vi "Get Column Object.vi"(8 "error in (no error)":errorcluster, 10 "Column Name":string, 11 "Table in":refnum<class "Table.lvclass">) -> (0 "error out":errorcluster, 2 "Column Object":refnum<class "Column Interface.lvclass">, 3 "Table out":refnum<class "Table.lvclass">)   [LabVIEW 2020, in "Table.lvlib" / "Table.lvclass"]
uses:
  Table.lvclass
  Column Interface/Column Interface Class/Column Interface.lvclass
  Table.lvclass/Table.ctl
  Table Configuration Interface/Table Configuration Interface.lvclass
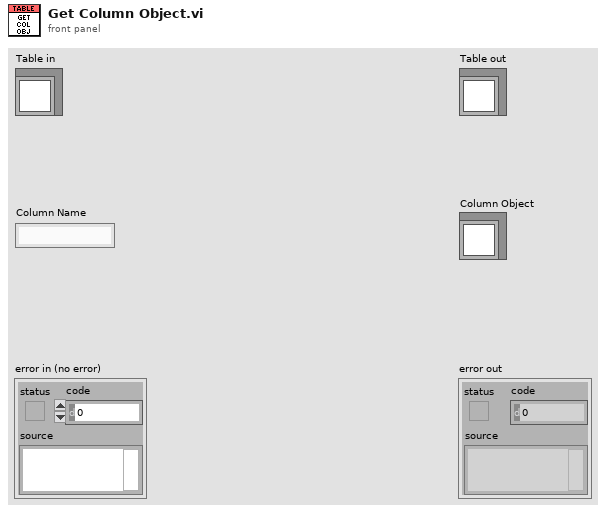
[diagram p1: front panel]
types:
  T1 = map{string, refnum<class "Column Interface.lvclass">}
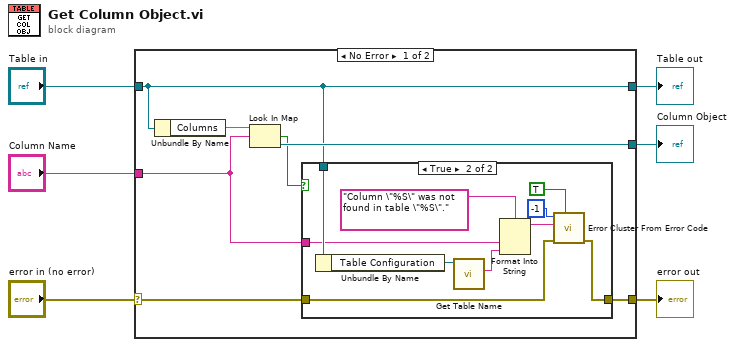
[diagram p0: block diagram]
diagram:
  n1 = case shown="No Error" "error in (no error)" {
    selector: "error in (no error)" -> [w8 w26]
    tunnel: [w7 w26] -> w5
    tunnel: [w11 w25] -> w3
    tunnel: "Table in" -> [w11 w25]
    tunnel: "Column Name" -> [w9 _]
    tunnel: [w12 _] -> w1
    frame No Error {
      n2 = Unbundle By Name(w11) -> ("Columns"=w13:T1)
      n3 = Look In Map(map=w13, key=w9) -> (key not found?=w10:bool, value=w12:refnum<class "Column Interface.lvclass">)  [unwired: 1 in]
      n4 = case shown="True" w10 {
        tunnel: w11 -> [_ w23]
        tunnel: w9 -> [_ w21]
        tunnel: [w14 w16] -> w7
        tunnel: w8 -> [w14 w15]
        frame False {
        }
        frame True {
          n5 = Unbundle By Name(w23) -> ("Table Configuration"=w22:refnum<class "Table Configuration Interface.lvclass">)
          n6 = call-dynamic "Get Table Name.vi"("Table Configuration Interface in"=w22) -> ("Table Name"=w20:string)  [unwired: 8 in, 2 out]
          n7 = Format Into String(format string="Column \"%S\" was not found in table \"%S\".", w21, w20) -> (resulting string=w19:string)  [unwired: 2 in, 1 out]
          n8 = call <vilib>:"Error Cluster From Error Code.vi"("show call chain? (False)"=TRUE, "error in (no error)"=w15, "error message (\"\")"=w19, "error code (0)"=-1) -> ("error out"=w16:errorcluster)  [unwired: 5 in]
        }
      }
    }
    frame Error {
    }
  }
  "error out" <- w5
  "Table out" <- w3
  "Column Object" <- w1
